vi "HW Run.vi"(8 "error in (no error)":errorcluster, 11 "ClusterOut in":T1) -> (0 "error out":errorcluster, 3 "ClusterOut out":T1)   [LabVIEW 2018]
uses:
  Queue/DataQueueElements.ctl
  Controls/Enums/TargetNumber.ctl
  Controls/Clusts/AcqData.ctl
  <vilib>/rvi/interface/nirviMethod/nirviMethod.xnode
  <vilib>/FPGAPlugInAG/Dynamic/niLvFpga_ReadFifo_Dynamic.vi
  <vilib>/rvi/errors/niLvFpgaMergeErrorWithErrorCode.vi
  Controls/Clusts/TimeDomainData.ctl
  Controls/Enums/LogLoopEnum.ctl
  Controls/Clusts/SaturationMonitor.ctl
  Controls/Clusts/FromFPGA_Clust.ctl
  Controls/Clusts/FPGA_Config_Clust.ctl
  Controls/HWCluster.ctl
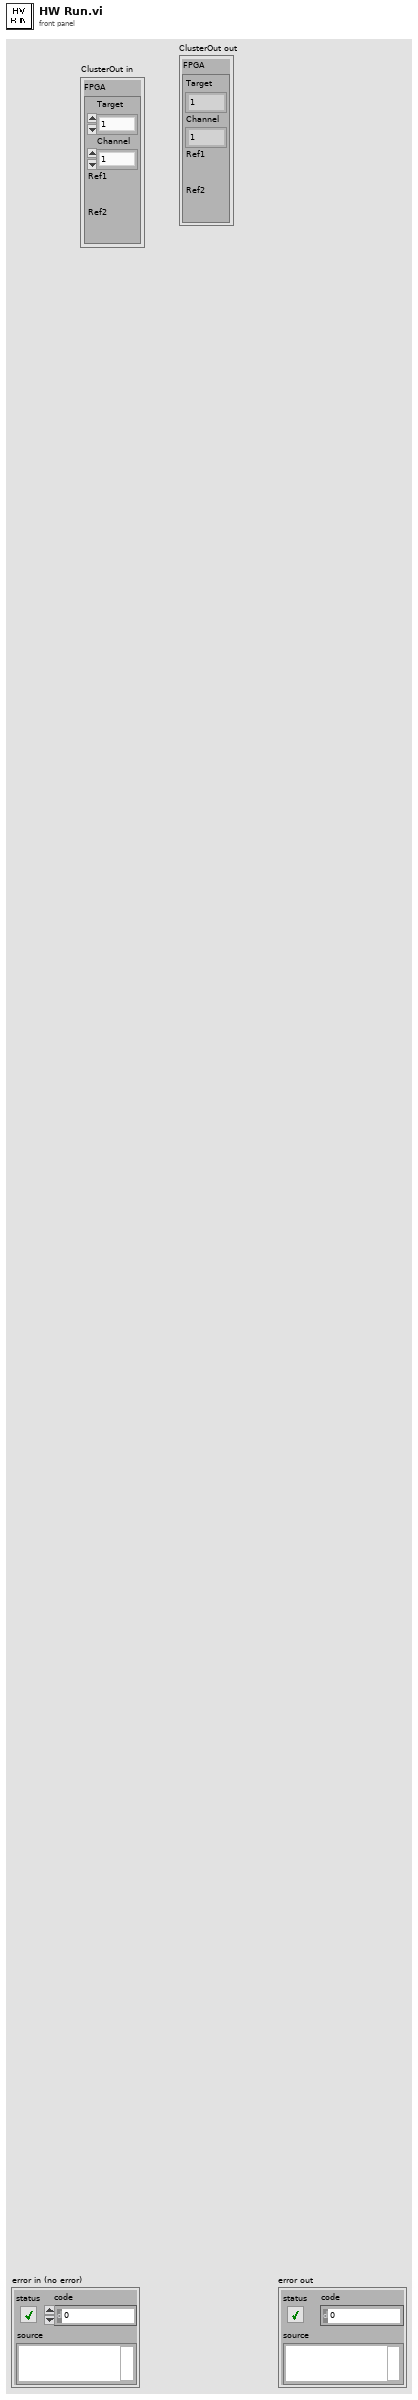
[diagram p1: front panel]
types:
  T1 = typedef "HWCluster.ctl" = cluster{"FPGA":T2}
  T2 = typedef "FPGA_Config_Clust.ctl" = cluster{"Target":T3, "Channel":T3, "Ref1":refnum<k20>, "Ref2":refnum<k20>}
  T3 = typedef "TargetNumber.ctl" = enum16{"1", "2", "3", "4"}
  T4 = typedef "DataQueueElements.ctl" = enum16{"Data_Init", "Data_Config", "Data_AddData", "Data_FreqShift", "Data_FPGA_Write", "Data_Transform", "Data_Send", "Data_Exit"}
  T5 = typedef "AcqData.ctl" = cluster{"Data":fxp<+/-,24,1>[], "#":T3, "Saturat":T6, "FromFPGA":T7, "10MHz":bool}
  T6 = typedef "SaturationMonitor.ctl" = cluster{"MeasMean0":dbl, "MeasMean1":dbl, "MeasMax":dbl, "1_Max":dbl, "4_Max":dbl, "5_Max":dbl, "6_Max":dbl, "7_Max":dbl}
  T7 = typedef "FromFPGA_Clust.ctl" = cluster{"CalTimeDomainI":ext[], "CalTimeDomainI.Index":ext[], "CalTimeDomainQ":ext[], "CalTimeDomainQ.Index":ext[], "BeacTimeDomainI":ext[], "BeacTimeDomainI.Index":ext[], "BeacTimeDomainQ":ext[], "BeacTimeDomainQ.Index":ext[]}
  T8 = typedef "LogLoopEnum.ctl" = enum16{"Log_Init", "Log_Config", "Log_CfgAlarm", "Log_TimeDomain", "Log_Tone", "Log_NoiseTrace", "Log_NoiseSum", "Log_DO", "Log_AI", "Log_TC", "Log_Disdrom", "Log_Weather", "Log_TE", "Log_ADAM", "Log_UPS", "Log_ChkTime", "Log_Alarm", "Log_Write", "Log_Exit"}
  T9 = typedef "TimeDomainData.ctl" = cluster{"CalTimeVal":dbl[], "CalTimeCount":u32[], "Enum":T3}
  T10 = cluster{"Data":ext[], ext, cluster{"MeasMean0":ext, "MeasMean1":ext, "MeasMax":ext, "1_Max":ext, "4_Max":ext, "5_Max":ext, "6_Max":ext, "7_Max":ext}, "FromFPGA":T7, "10MHz":ext}
  T11 = typedef "Semaphore RefNum" = refnum<k1>
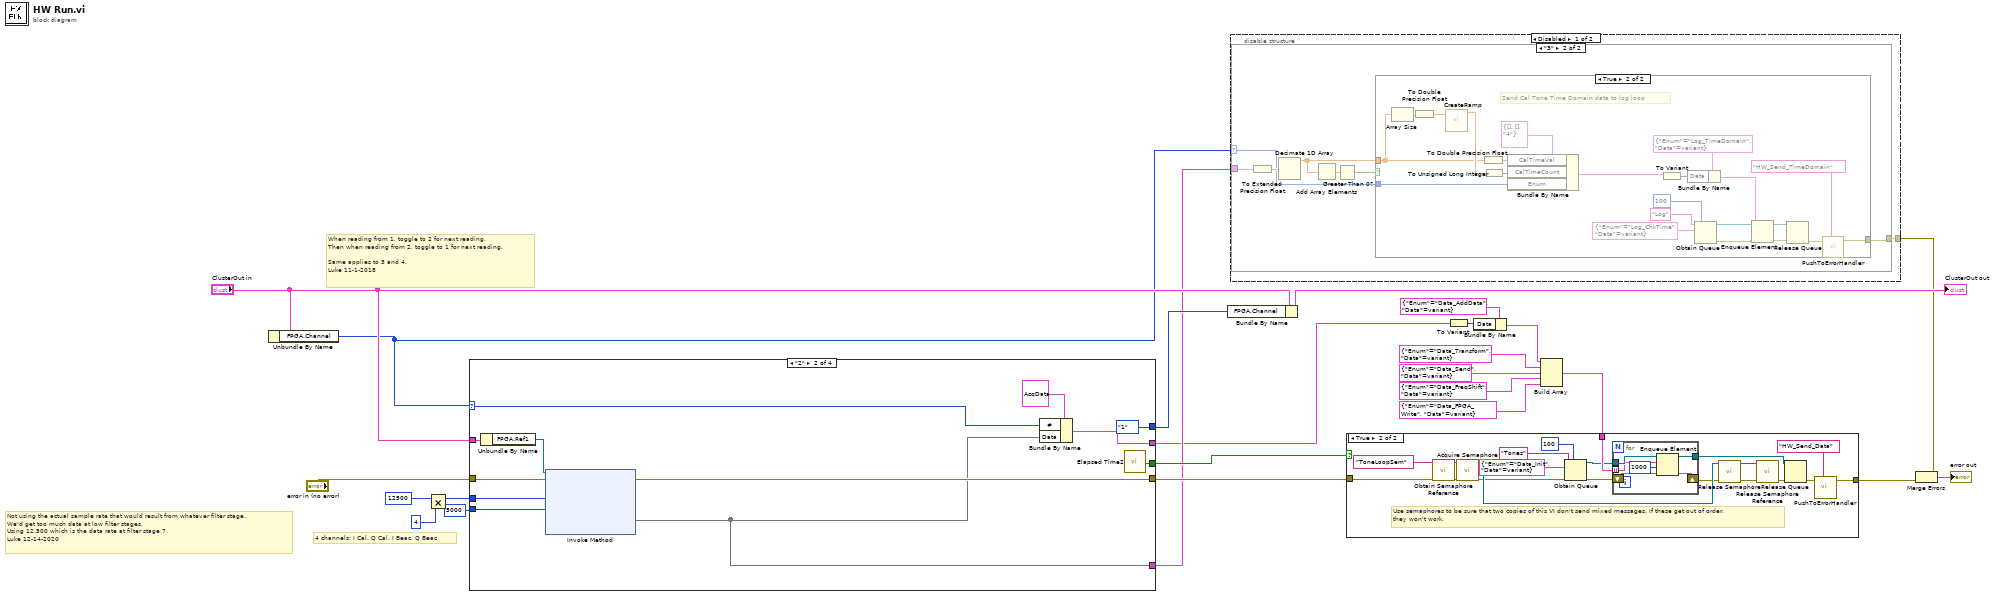
[diagram p0: block diagram]
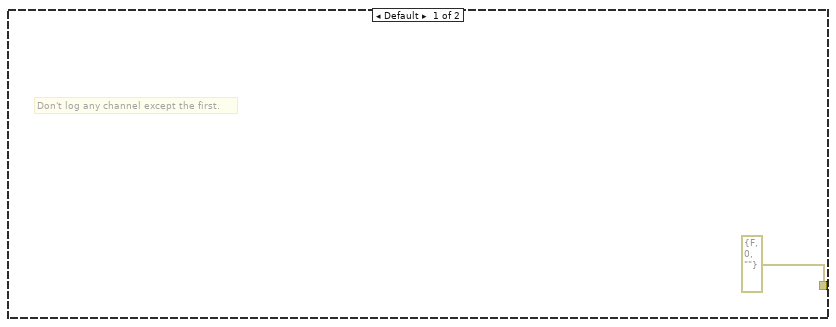
[diagram p2: hidden frame]
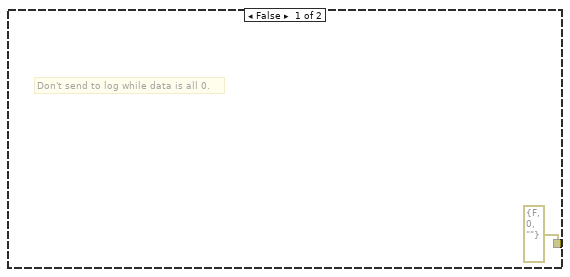
[diagram p3: hidden frame]
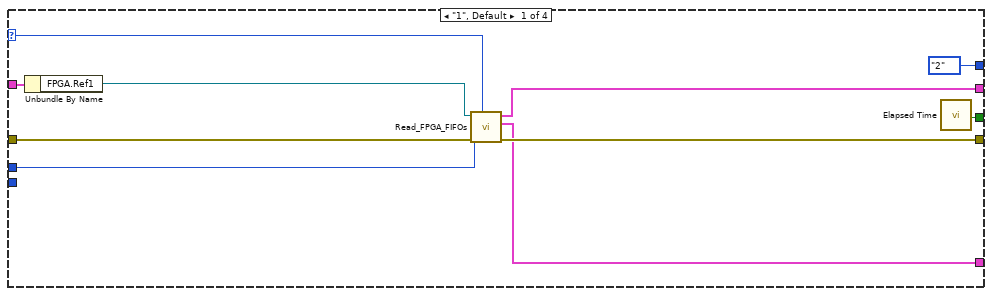
[diagram p6: hidden frame]
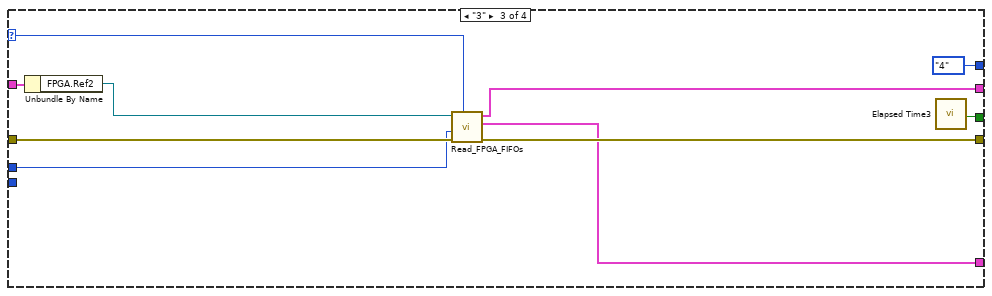
[diagram p7: hidden frame]
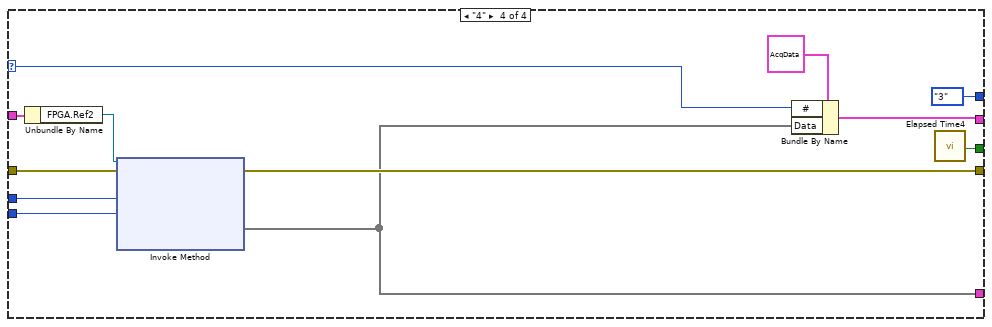
[diagram p8: hidden frame]
diagram:
  # "Not using the actual sample rate that would result from whatever filter stage.\nWe'd get too much data at low filter stages.\nUsing 12,500 which is the data rate at filter stage 7.\nLuke 12-14-2020"
  # "4 channels: I Cal, Q Cal, I Beac, Q Beac"
  # "When reading from 1, toggle to 2 for next reading.\nThen when reading from 2, toggle to 1 for next reading.\n\nSame applies to 3 and 4. \nLuke 11-1-2018"
  n1 = Unbundle By Name("ClusterOut in") -> ("FPGA.Channel"=w5:T3)
  n2 = Multiply(x=u32 12500, y=u32 4) -> (x*y=w8:u32)
  n3 = case shown="\"2\"" w5 {
    selector: w5 -> [w25 w35 w50 w58]
    tunnel: w8 -> [w34 w46 w49 w68]
    tunnel: 5000 ("Timeout (ms)") -> [_ w45 _ w67]
    tunnel: "error in (no error)" -> [w33 w44 w53 w66]
    tunnel: [w27 w36 w48 w57] -> w6
    tunnel: [w28 w43 w52 w65] -> w19
    tunnel: "ClusterOut in" -> [w32 w41 w56 w63]
    tunnel: [TargetNumber."2" ("FPGA.Target") TargetNumber."1" ("FPGA.Target") TargetNumber."4" ("FPGA.Target") TargetNumber."3" ("FPGA.Target")] -> w23
    tunnel: [w30 w39 w54 w61] -> w24
    tunnel: [w26 w37 w47 w59] -> w2
    frame "1", Default {
      n4 = Unbundle By Name(w32) -> ("FPGA.Ref1"=w29:refnum<k20>)
      n5 = call "Read_FPGA_FIFOs.vi"("TargetA"=w25, "error in"=w33, "#Elements"=w34, "FPGA VI Ref"=w29) -> ("error out"=w28:errorcluster, "AcqDataB"=w27:T5, "AcqDataA"=w26:T5)  [unwired: 4 in, 1 out]
      n6 = call "Elapsed Time"() -> ("Time has Elapsed"=w30:bool)  [unwired: 12 in, 7 out]
    }
    frame "2" {
      n7 = Unbundle By Name(w41) -> ("FPGA.Ref1"=w42:refnum<k20>)
      n8 = xnode "Invoke Method"("FPGA VI Reference In"=w42, "error in"=w44, "Number of Elements"=w46, "Timeout (ms)"=w45) -> ("error out"=w43:errorcluster, "Data"=w36:void[])  [unwired: 2 out]
      n9 = Bundle By Name(cluster=T5 {"Data"=[], "#"=enum."1", "Saturat"={"MeasMean0"=0.0, "MeasMean1"=0.0, "MeasMax"=0.0, "1_Max"=0.0, "4_Max"=0.0, "5_Max"=0.0, "6_Max"=0.0, "7_Max"=0.0}, "FromFPGA"={"CalTimeDomainI"=[], "CalTimeDomainI.Index"=[], "CalTimeDomainQ"=[], "CalTimeDomainQ.Index"=[], "BeacTimeDomainI"=[], "BeacTimeDomainI.Index"=[], "BeacTimeDomainQ"=[], "BeacTimeDomainQ.Index"=[]}, "10MHz"=FALSE}, "#"=w35, "Data"=w36) -> (w37:T5)
      n10 = call "Elapsed Time2"() -> ("Time has Elapsed"=w39:bool)  [unwired: 12 in, 7 out]
    }
    frame "3" {
      n11 = Unbundle By Name(w56) -> ("FPGA.Ref2"=w51:refnum<k20>)
      n12 = call "Read_FPGA_FIFOs.vi"("TargetA"=w50, "error in"=w53, "#Elements"=w49, "FPGA VI Ref"=w51) -> ("error out"=w52:errorcluster, "AcqDataB"=w48:T5, "AcqDataA"=w47:T5)  [unwired: 4 in, 1 out]
      n13 = call "Elapsed Time3"() -> ("Time has Elapsed"=w54:bool)  [unwired: 12 in, 7 out]
    }
    frame "4" {
      n14 = Unbundle By Name(w63) -> ("FPGA.Ref2"=w64:refnum<k20>)
      n15 = xnode "Invoke Method"("FPGA VI Reference In"=w64, "error in"=w66, "Number of Elements"=w68, "Timeout (ms)"=w67) -> ("error out"=w65:errorcluster, "Data"=w57:void[])  [unwired: 2 out]
      n16 = Bundle By Name(cluster=T5 {"Data"=[], "#"=enum."1", "Saturat"={"MeasMean0"=0.0, "MeasMean1"=0.0, "MeasMax"=0.0, "1_Max"=0.0, "4_Max"=0.0, "5_Max"=0.0, "6_Max"=0.0, "7_Max"=0.0}, "FromFPGA"={"CalTimeDomainI"=[], "CalTimeDomainI.Index"=[], "CalTimeDomainQ"=[], "CalTimeDomainQ.Index"=[], "BeacTimeDomainI"=[], "BeacTimeDomainI.Index"=[], "BeacTimeDomainQ"=[], "BeacTimeDomainQ.Index"=[]}, "10MHz"=FALSE}, "#"=w58, "Data"=w57) -> (w59:T5)
      n17 = call "Elapsed Time4"() -> ("Time has Elapsed"=w61:bool)  [unwired: 12 in, 7 out]
    }
  }
  n18 = Bundle By Name(cluster="ClusterOut in", "FPGA.Channel"=w23) -> (→"ClusterOut out":T1)
  n19 = disable-structure shown="Disabled" {
    disable-tunnel: w6 -> [w71 _]
    disable-tunnel: w5 -> [w70 _]
    disable-tunnel: [w69 _] -> w3
    frame Disabled {
      n20 = case shown="\"3\"" w70 {
        selector: w70 -> [_ w78]
        tunnel: w71 -> [_ w77]
        tunnel: [errorcluster {"status"=FALSE, "code"=0, "source"=""} ("ErrorOut") w76] -> w69
        frame Default {
          # "Don't log any channel except the first."
        }
        frame "3" {
          n21 = To Extended Precision Float(1:w77) -> (0:w79:T10)
          n22 = Decimate 1D Array(w79) -> (w73:dbl[])  [unwired: 3 out]
          n23 = Add Array Elements(numeric array=w73) -> (sum=w75:dbl)
          n24 = Greater Than 0?(x=w75) -> (x > 0?=w74:bool)
          n25 = case shown="True" w74 {
            tunnel: w78 -> [_ w100]
            tunnel: [errorcluster {"status"=FALSE, "code"=0, "source"=""} ("ErrorOut") w83] -> w76
            tunnel: w73 -> [_ w81]
            frame False {
              # "Don't send to log while data is all 0."
            }
            frame True {
              # "Send Cal Tone Time Domain data to log loop"
              n26 = Array Size(array=w81) -> (size(s)=w98:i32)
              n27 = To Double Precision Float(number=w98) -> (double precision float=w96:dbl)
              n28 = call "CreateRamp.vi"("ArraySize"=w96) -> ("Ramp Pattern"=w97:dbl[])  [unwired: 10 in]
              n29 = To Double Precision Float(number=w81) -> (double precision float=w101:dbl[])
              n30 = To Unsigned Long Integer(number=w97) -> (unsigned 32bit integer=w99:u32[])
              n31 = Bundle By Name(cluster=T9 {"CalTimeVal"=[], "CalTimeCount"=[], "Enum"=enum."4"} ("TimeDomain"), "CalTimeVal"=w101, "CalTimeCount"=w99, "Enum"=w100) -> (w88:T9)
              n32 = To Variant(anything=w88) -> (Variant=w89:variant)
              n33 = Bundle By Name(cluster=cluster{"Enum":T8, "Data":variant} {"Enum"=enum."Log_TimeDomain", "Data"=variant} ("element"), "Data"=w89) -> (w90:cluster{"Enum":T8, "Data":variant})
              n34 = Obtain Queue(max queue size (-1, unlimited)=100, name (unnamed)="Log", element data type=cluster{"Enum":T8, "Data":variant} {"Enum"=enum."Log_ChkTime", "Data"=variant}) -> (queue out=w93:refnum<queue>, error out=w87:errorcluster)  [unwired: 2 in, 1 out]
              n35 = Enqueue Element(queue=w93, element=w90, error in (no error)=w87) -> (queue out=w86:refnum<queue>, error out=w85:errorcluster)  [unwired: 1 in, 1 out]
              n36 = Release Queue(queue=w86, error in (no error)=w85) -> (error out=w84:errorcluster)  [unwired: 1 in, 2 out]
              n37 = call "PushToErrorHandler.vi"("ErrorIn"=w84, "ErrorLocation"="HW_Send_TimeDomain") -> ("ErrorOut"=w83:errorcluster)  [unwired: 5 in]
            }
          }
        }
      }
    }
    frame Enabled {
    }
  }
  n38 = To Variant(anything=w2) -> (Variant=w13:variant)
  n39 = Bundle By Name(cluster=cluster{"Enum":T4, "Data":variant} {"Enum"=enum."Data_AddData", "Data"=variant}, "Data"=w13) -> (w12:cluster{"Enum":T4, "Data":variant})
  n40 = Build Array(w12, cluster{"Enum":T4, "Data":variant} {"Enum"=enum."Data_Transform", "Data"=variant}, cluster{"Enum":T4, "Data":variant} {"Enum"=enum."Data_Send", "Data"=variant}, cluster{"Enum":T4, "Data":variant} {"Enum"=enum."Data_FreqShift", "Data"=variant}, cluster{"Enum":T4, "Data":variant} {"Enum"=enum."Data_FPGA_Write", "Data"=variant}) -> (w18:cluster{"Enum":T4, "Data":variant}[])
  n41 = case shown="True" w24 {
    tunnel: w18 -> [_ w115]
    tunnel: w19 -> [w103 w111]
    tunnel: [w103 w105] -> w20
    frame False {
      # "If decimation stages are turned off (on main front panel on 'filter scaling' tab) data comes from FPGA too quickly\nfor data/tones loop to keep up. We have to throttle the data here to prevent lags.\nLuke 2-11-2019"
    }
    frame True {
      # "Use semaphores to be sure that two copies of this VI don't send mixed messages. If these get out of order,\nthey won't work."
      n42 = call <vilib>:"Obtain Semaphore Reference.vi"("error in (no error)"=w111, "name (unnamed)"="ToneLoopSem") -> ("error out"=w118:errorcluster, "semaphore"=w120:T11)  [unwired: 3 in, 1 out]
      n43 = call <vilib>:"Acquire Semaphore.vi"("error in (no error)"=w118, "semaphore"=w120) -> ("error out"=w110:errorcluster, "semaphore out"=w119:T11)  [unwired: 3 in, 1 out]
      n44 = Obtain Queue(max queue size (-1, unlimited)=100, name (unnamed)="Tones", element data type=cluster{"Enum":T4, "Data":variant} {"Enum"=enum."Data_Init", "Data"=variant}, error in (no error)=w110) -> (queue out=w114:refnum<queue>, error out=w109:errorcluster)  [unwired: 1 in, 1 out]
      n45 = for {
        tunnel: w114 -> [w127]
        tunnel: w115 -> [w126] mode=indexing
        shift-right: [w128] -> w116
        shift-left: w109 -> [w129]
        tunnel: [w125] -> w107
        n46 = Enqueue Element(queue=w127, element=w126, timeout in ms (-1)=1000, error in (no error)=w129) -> (queue out=w125:refnum<queue>, error out=w128:errorcluster)  [unwired: 1 out]
      }
      n47 = call <vilib>:"Release Semaphore.vi"("error in (no error)"=w116, "semaphore"=w119) -> ("error out"=w117:errorcluster, "semaphore out"=w113:T11)  [unwired: 4 in]
      n48 = call <vilib>:"Release Semaphore Reference.vi"("error in (no error)"=w117, "semaphore"=w113) -> ("error out"=w108:errorcluster)  [unwired: 8 in, 1 out]
      n49 = Release Queue(queue=w107, error in (no error)=w108) -> (error out=w106:errorcluster)  [unwired: 1 in, 2 out]
      n50 = call "PushToErrorHandler.vi"("ErrorIn"=w106, "ErrorLocation"="HW_Send_Data") -> ("ErrorOut"=w105:errorcluster)  [unwired: 5 in]
    }
  }
  n51 = Merge Errors(w3, w20) -> (→"error out":errorcluster)
